vi "rad_Retrieve SysCfg AppImage Properties from Target.vi"(5 "Password":string, 8 "error in (no error)":errorcluster, 11 "Target settings":T1={"Hostname"="", "Serial number"="", "Product name"="", "Product code"=0, "System status"="", "Credential type"=enum."None/Unlocked", "User added?"=FALSE, "Primary NIC"={"MAC address"="", "IP Address Request Mode"=2, "IP address"="", "Subnet mask"="", "Gateway"="", "DNS server"=""}} {"Primary NIC"."IP Address Request Mode" items=["Static"=1, "DHCP/Link-Local"=2, "Link-Local Only"=4, "DHCP Only"=8]}) -> (0 "error out":errorcluster, 2 "Supports System\nConfig Metadata":bool, 3 "image metadata":T3={"title"="", "description"="", "ID"="", "version"="", "component type"=5} {"component type" items=["standard", "hidden", "system", "unknown", "startup", "image"]})   [LabVIEW 2020]
uses:
  <resource>/objmgr/nisysapi.rc
  <vilib>/nisyscfg/nisyscfg.lvlib
  <vilib>/nisyscfg/Close (System).vi
  <vilib>/nisyscfg/Software 1.2.ctl
  <vilib>/nisyscfg/Component Type.ctl
  Targets/TypeDefs/rad_Target Information.ctl
  Targets/TypeDefs/rad_Target Network Settings.ctl
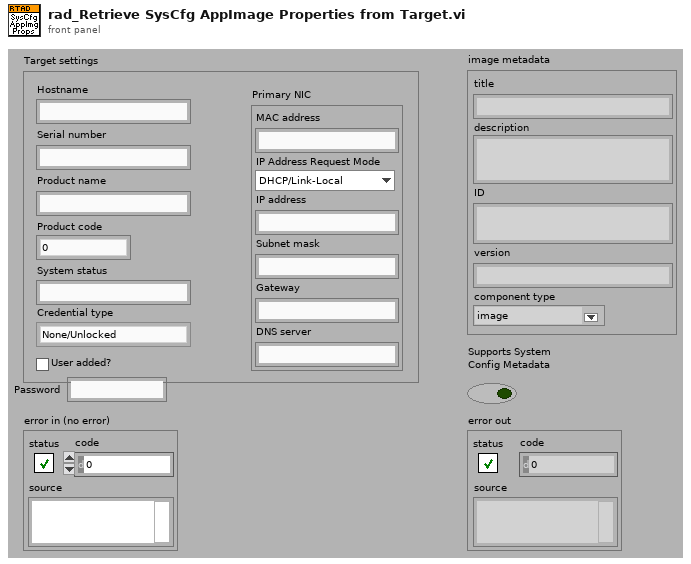
[diagram p1: front panel]
types:
  T1 = typedef "rad_Target Information.ctl" = cluster{"Hostname":string, "Serial number":string, "Product name":string, "Product code":i32, "System status":string, "Credential type":enum16{"None/Unlocked", "FTP Password", "NIAuth Credentials"}, "User added?":bool, "Primary NIC":T2}
  T2 = typedef "rad_Target Network Settings.ctl" = cluster{"MAC address":string, "IP Address Request Mode":i32, "IP address":string, "Subnet mask":string, "Gateway":string, "DNS server":string}
  T3 = typedef "nisyscfg.lvlib/Software 1.2.ctl" = cluster{"title":string, "description":string, "ID":string, "version":string, "component type":T4}
  T4 = typedef "nisyscfg.lvlib/Component Type.ctl" = u32
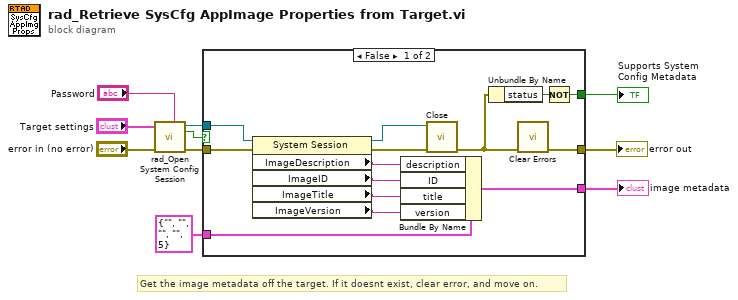
[diagram p0: block diagram]
diagram:
  # "Get the image metadata off the target. If it doesnt exist, clear error, and move on."
  n1 = call "rad_Open System Config Session.vi"("Password"="Password", "error in (no error)"="error in (no error)", "Target settings"="Target settings") -> ("error out"=w5:errorcluster, "Cancelled"=w6:bool, "Session out"=w7:refnum<k21>)  [unwired: 5 in, 1 out]
  n2 = case shown="False" w6 {
    tunnel: w7 -> [w24 _]
    tunnel: w5 -> [w23 w26]
    tunnel: [w15 w26] -> w9
    tunnel: [w17 w25] -> w8
    tunnel: T3 {"title"="", "description"="", "ID"="", "version"="", "component type"=5} ("image metadata") -> [w16 w25]
    tunnel: [w11 _] -> w2
    frame False {
      n3 = property class="System Session"(reference=w24, error in=w23) -> (reference out=w18:refnum<k21>, error out=w19:errorcluster, "ImageDescription"=w22:string, "ImageID"=w14:string, "ImageTitle"=w21:string, "ImageVersion"=w20:string)
      n4 = Bundle By Name(cluster=w16, "description"=w22, "ID"=w14, "title"=w21, "version"=w20) -> (w17:T3)
      n5 = call-poly <vilib>:"Close.vi"("error in (no error)"=w19, "Session in"=w18) -> ("error out"=w13:errorcluster)  [unwired: 9 in]
      n6 = Unbundle By Name(w13) -> ("status"=w12:bool)
      n7 = call <vilib>:"Clear Errors.vi"("error in (no error)"=w13) -> ("error out"=w15:errorcluster)  [unwired: 5 in, 1 out]
      n8 = Not(x=w12) -> (.not. x?=w11:bool)
    }
    frame True {
    }
  }
  "image metadata" <- w8
  "error out" <- w9
  "Supports System\nConfig Metadata" <- w2
